vi "I2C_Send_1_Bit_DAQ.vi"(2 "Data_Bit":bool) -> ()   [LabVIEW 2022 SP3]
doc: "Petrus Prins 7 June 2026"
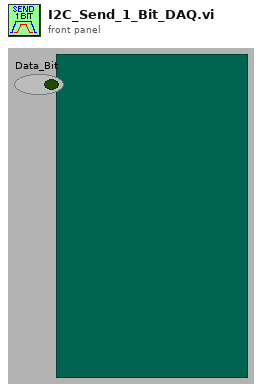
[diagram p1: front panel]
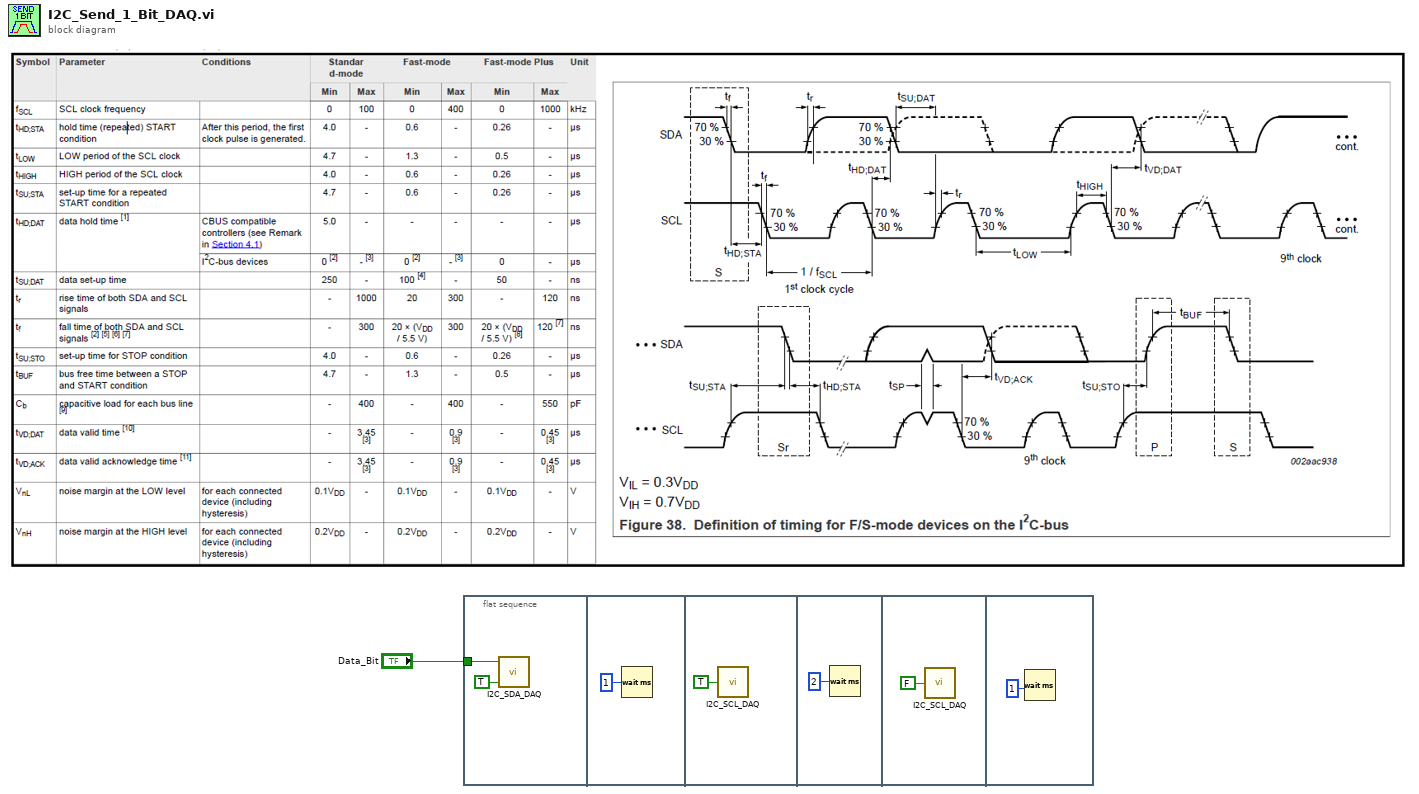
[diagram p0: block diagram]
diagram:
  n1 = flat-sequence {
    tunnel: "Data_Bit" -> [w3]
    frame #0 {
      n2 = call "I2C_SDA_DAQ.vi"("Tx_or_Rx?"=TRUE, "Tx_Data"=w3) -> ()  [unwired: 1 in, 1 out]
    }
    frame #1 {
      n3 = Wait (ms)(milliseconds to wait=u32 1) -> ()  [unwired: 1 out]
    }
    frame #2 {
      n4 = call "I2C_SCL_DAQ.vi"("SCL_Data"=TRUE) -> ()  [unwired: 5 in]
    }
    frame #3 {
      n5 = Wait (ms)(milliseconds to wait=u32 2) -> ()  [unwired: 1 out]
    }
    frame #4 {
      n6 = call "I2C_SCL_DAQ.vi"("SCL_Data"=FALSE) -> ()  [unwired: 5 in]
    }
    frame #5 {
      n7 = Wait (ms)(milliseconds to wait=u32 1) -> ()  [unwired: 1 out]
    }
  }
